vi "Append Row to Traces.vi"(8 "error in (no error)":errorcluster, 10 "Trace.lvclass":refnum<class "Trace.lvclass">, 11 "Tracer-V in":refnum<class "Tracer-V.lvclass">) -> (0 "error out":errorcluster, 3 "Tracer-V out":refnum<class "Tracer-V.lvclass">)   [LabVIEW 2013, in "Tracer-V.lvclass"]
uses:
  Tracer-V.lvclass
  Logical Systems/TraceMessage/Trace.lvclass
  Tracer-V.lvclass/Tracer-V.ctl
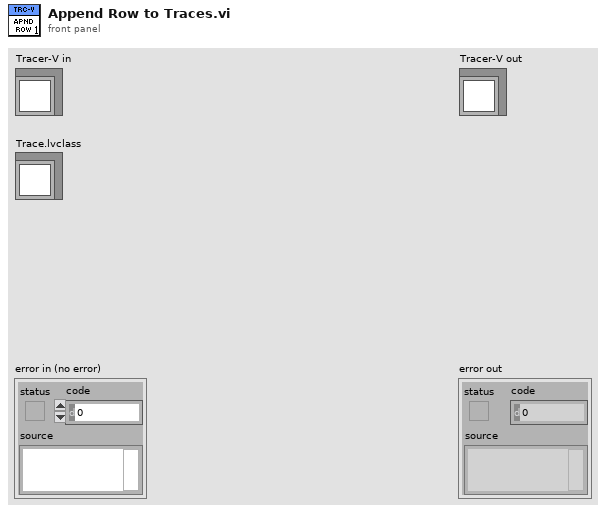
[diagram p1: front panel]
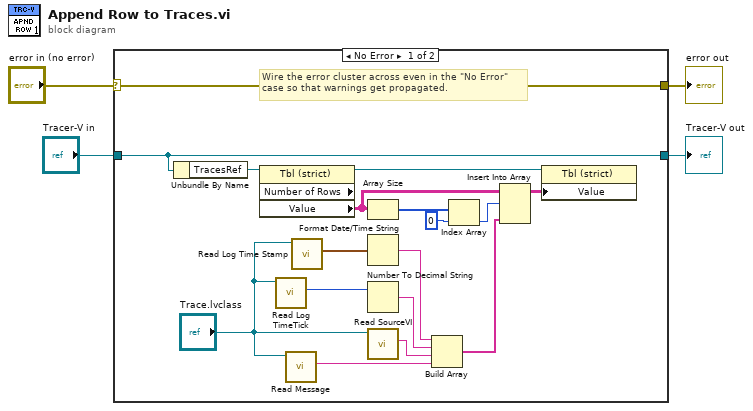
[diagram p0: block diagram]
diagram:
  n1 = case shown="No Error" "error in (no error)" {
    selector: "error in (no error)" -> [w21 w23]
    tunnel: [w21 w23] -> w3
    tunnel: [w20 w22] -> w1
    tunnel: "Tracer-V in" -> [w20 w22]
    frame No Error {
      # "Wire the error cluster across even in the \"No Error\"\ncase so that warnings get propagated."
      n2 = Unbundle By Name(w20) -> ("TracesRef"=w19:refnum<vi>)
      n3 = property class="Tbl (strict)" props=["Number of Rows", "Value"](reference=w19) -> (reference out=w18:refnum<vi>, "Value"=w15:string[][])  [unwired: 1 in, 2 out]
      n4 = call-dynamic "Read Log TimeTick.vi"("TraceMessage in"="Trace.lvclass") -> ("Trace TimeTick"=w9:u32)  [unwired: 8 in, 2 out]
      n5 = call-dynamic "Read Message.vi"("TraceMessage in"="Trace.lvclass") -> ("Message"=w6:string)  [unwired: 8 in, 2 out]
      n6 = call-dynamic "Read Log Time Stamp.vi"("Trace in"="Trace.lvclass") -> ("Log Time Stamp"=w17:timestamp)  [unwired: 8 in, 2 out]
      n7 = Array Size(array=w15) -> (size(s)=w14:i32[])
      n8 = Format Date/Time String(seconds (now)=w17) -> (date/time string=w16:string)  [unwired: 2 in]
      n9 = Number To Decimal String(number=w9) -> (decimal integer string=w8:string)  [unwired: 1 in]
      n10 = call-dynamic "Read SourceVI.vi"("Trace in"="Trace.lvclass") -> ("SourceVI"=w7:string)  [unwired: 8 in, 2 out]
      n11 = Build Array(w16, w8, w7, w6) -> (w11:string[])
      n12 = Index Array(array=w14, index=0) -> (element=w12:i32)
      n13 = Insert Into Array(array=w15, index (row)=w12, new element=w11) -> (w10:string[][])  [unwired: 1 in]
      n14 = property class="Tbl (strict)"(reference=w18, "Value"=w10) -> ()  [unwired: 1 in, 2 out]
    }
    frame Error {
    }
  }
  "error out" <- w3
  "Tracer-V out" <- w1
